vi "Cluster Terminal Get Elements Info.vi"(7 "skip first typedef?":bool, 8 "error in (no error)":errorcluster, 10 "ClusterConstant refnum":refnum<vi>, 11 "Terminal in":refnum<vi>) -> (0 "error out":errorcluster, 1 "is typedef?":bool, 2 "Cluster elements datatypes":string[](array[string]), 3 "Cluster elements names":string[](array[string]), 4 "typedef name":string)   [LabVIEW 2014]
doc: "Return info about cluster elements, as input use Terminal or ClusterConstant (use just one of them)\nIf wired Cluster Constant refnum returns names and datatypes of elements inside cluster. If elemnet has no label, it's returned default name \"item0\" or \"item1\" or ... \"itemN\" which will be also used in generated code.\nIf wired Terminal then is used to get names and datatypes of cluster, it will programmaticaly creates cluster constant on diagram, inspects its elements, removes it and return elements info."
uses:
  TranscriptorBasicObject.lvclass
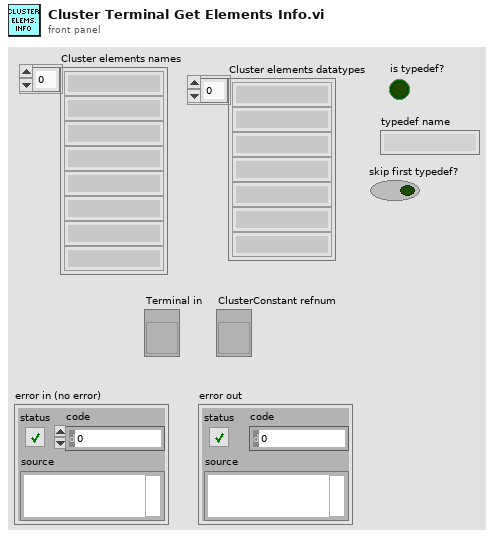
[diagram p1: front panel]
types:
  T1 = enum32{"not a typedef", "typedef", "strict typedef", "class private data"}[]
  T2 = enum32{"not a typedef", "typedef", "strict typedef", "class private data"}
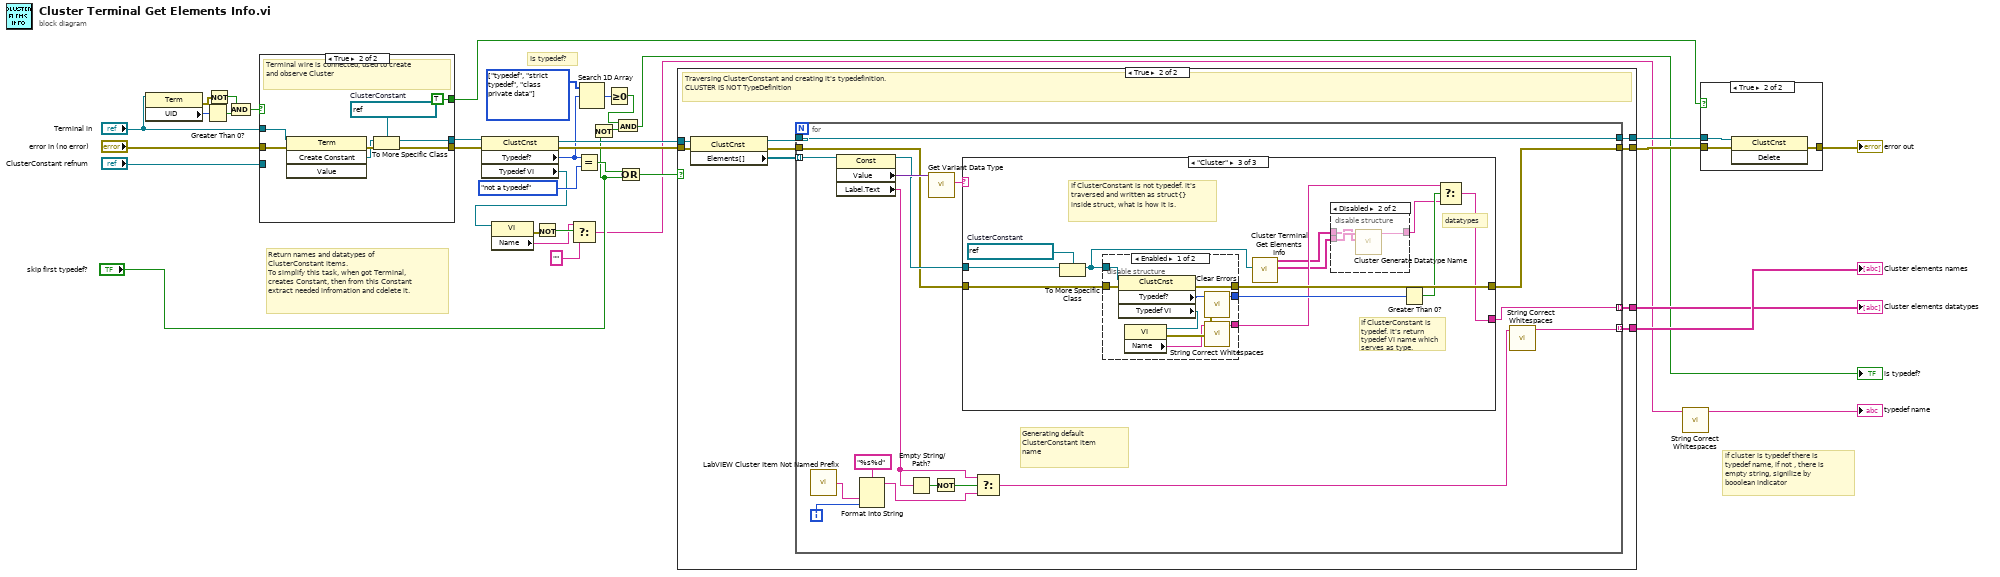
[diagram p0: block diagram]
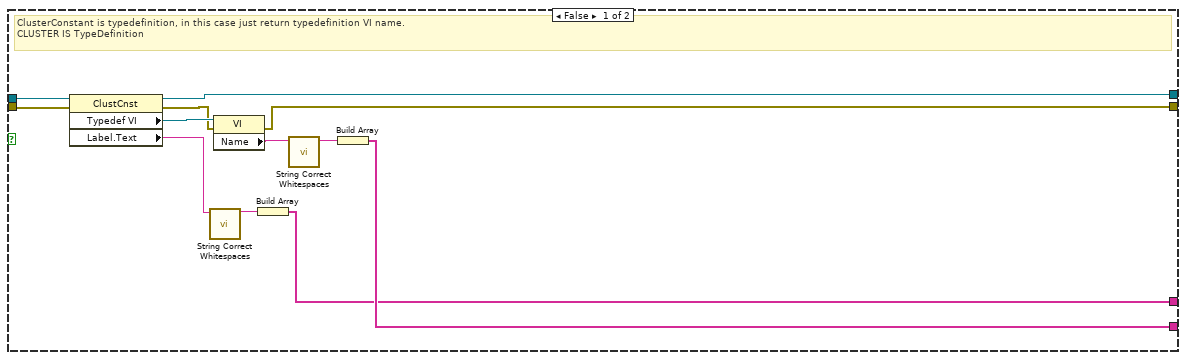
[diagram p2: hidden frame]
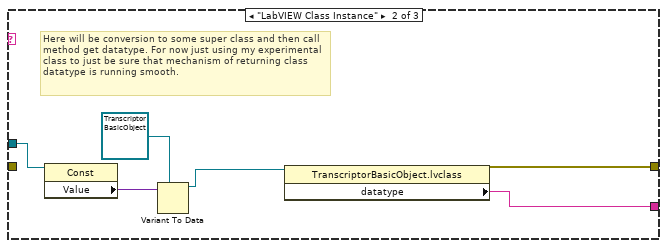
[diagram p4: hidden frame]
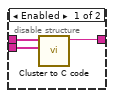
[diagram p5: hidden frame]
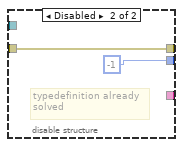
[diagram p6: hidden frame]
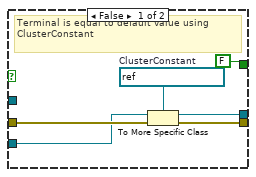
[diagram p8: hidden frame]
diagram:
  w16 = T1 [enum."typedef", enum."strict typedef", enum."class private data"] items=["not a typedef", "typedef", "strict typedef", "class private data"]
  # "if cluster is typedef there is typedef name, if not , there is empty string, signilize by booolean indicator"
  # "Is typedef?"
  # "Return names and datatypes of ClusterConstant items.\nTo simplify this task, when got Terminal, creates Constant, then from this Constant extract needed infromation and cdelete it."
  n1 = property class="Term"(reference="Terminal in") -> (error out=w20:errorcluster, "UID"=w22:i32)  [unwired: 1 in, 1 out]
  n2 = Greater Than 0?(x=w22) -> (x > 0?=w21:bool)
  n3 = Not(x=w20) -> (.not. x?=w19:bool)
  n4 = And(x=w19, y=w21) -> (x .and. y?=w18:bool)
  n5 = case shown="True" w18 {
    tunnel: [w39 w49] -> w28
    tunnel: "error in (no error)" -> [w38 w47]
    tunnel: [w40 w45] -> w29
    tunnel: "Terminal in" -> [_ w43]
    tunnel: [FALSE TRUE] -> w25
    tunnel: "ClusterConstant refnum" -> [w36 _]
    frame False {
      w41 = refnum<vi> refnum  # ClusterConstant
      # "Terminal is equal to default value using ClusterConstant"
      n6 = To More Specific Class(target class=w41, reference=w36, error in=w38) -> (specific class reference=w40:refnum<vi>, error out=w39:errorcluster)
    }
    frame True {
      w44 = refnum<vi> refnum  # ClusterConstant
      # "Terminal wire is connected, used to create and observe Cluster"
      n7 = invoke on="Invoke Node" class="Term" method="Create Constant"(reference=w43, error in=w47) -> (error out=w48:errorcluster, "Create Constant"=w46:refnum<vi>)  [unwired: 2 in, 2 out]
      n8 = To More Specific Class(target class=w44, reference=w46, error in=w48) -> (specific class reference=w45:refnum<vi>, error out=w49:errorcluster)
    }
  }
  n9 = property on="Property Node" class="ClustCnst"(reference=w29, error in=w28) -> (reference out=w27:refnum<vi>, error out=w26:errorcluster, "Typedef?"=w15:T2, "Typedef VI"=w7:refnum<vi>)
  n10 = property on="Property Node" class="VI"(reference=w7) -> (error out=w6:errorcluster, "Name"=w4:string)  [unwired: 1 in, 1 out]
  n11 = Not(x=w6) -> (.not. x?=w5:bool)
  n12 = Select(t=w4, s=w5, f="") -> (s? t:f=w2:string)
  n13 = Equal?(x=w15, y=T2."not a typedef" ("Is Typedef?")) -> (x = y?=w13:bool)
  n14 = Search 1D Array(1D array=w16, element=w15) -> (index of element=w14:i32)  [unwired: 1 in]
  n15 = Not(x="skip first typedef?") -> (.not. x?=w8:bool)
  n16 = Greater Or Equal To 0?(x=w14) -> (x >= 0?=w11:bool)
  n17 = And(x=w11, y=w8) -> (x .and. y?=→"is typedef?":bool)
  n18 = Or(x=w13, y="skip first typedef?") -> (x .or. y?=w12:bool)
  n19 = case shown="True" w12 {
    tunnel: [w55 w70] -> w34
    tunnel: w26 -> [w60 w68]
    tunnel: w27 -> [w61 w66]
    tunnel: [w57 w64] -> w32
    tunnel: [w53 w63] -> w31
    tunnel: [w52 w62] -> w30
    frame False {
      # "ClusterConstant is typedefinition, in this case just return typedefinition VI name.\nCLUSTER IS TypeDefinition"
      n20 = property on="Property Node" class="ClustCnst"(reference=w61, error in=w60) -> (reference out=w57:refnum<vi>, error out=w56:errorcluster, "Typedef VI"=w59:refnum<vi>, "Label.Text"=w51:string)
      n21 = call "String Correct Whitespaces.vi"("String in"=w51) -> ("String out"=w50:string)  [unwired: 10 in]
      n22 = property on="Property Node" class="VI"(reference=w59, error in=w56) -> (error out=w55:errorcluster, "Name"=w58:string)  [unwired: 1 out]
      n23 = Build Array(w50) -> (w52:string[])
      n24 = call "String Correct Whitespaces.vi"("String in"=w58) -> ("String out"=w54:string)  [unwired: 10 in]
      n25 = Build Array(w54) -> (w53:string[])
    }
    frame True {
      # "Traversing ClusterConstant and creating it's typedefinition.\nCLUSTER IS NOT TypeDefinition"
      n26 = property on="Property Node" class="ClustCnst"(reference=w66, error in=w68) -> (reference out=w65:refnum<vi>, error out=w69:errorcluster, "Elements[]"=w67:refnum<vi>[])
      n27 = for {
        tunnel: w67 -> [w87] mode=indexing
        tunnel: w69 -> [w71]
        tunnel: [w73] -> w70
        tunnel: w65 -> [w79]
        tunnel: [w79] -> w64
        tunnel: [w72] -> w62 mode=indexing
        tunnel: [w78] -> w63 mode=indexing
        i -> [w82]
        # "Generating default ClusterConstant item name"
        n28 = call "LabVIEW Cluster Item Not Named Prefix.vi"() -> ("not named cluster item prefix"=w81:string)
        n29 = property class="Const"(reference=w87) -> (reference out=w74:refnum<vi>, "Value"=w75:variant, "Label.Text"=w80:string)  [unwired: 1 in, 1 out]
        n30 = Format Into String(format string="%s%d", w81, w82) -> (resulting string=w83:string)  [unwired: 2 in, 1 out]
        n31 = Empty String/Path?(string/path=w80) -> (empty?=w86:bool)
        n32 = call "Get Variant Data Type.vi"("Variant in"=w75) -> ("first data type"=w76:string)  [unwired: 9 in, 1 out]
        n33 = Not(x=w86) -> (.not. x?=w85:bool)
        n34 = case shown="\"Cluster\"" w76 {
          selector: w76 -> [w88 _ _]
          tunnel: w74 -> [_ w93 w96]
          tunnel: w71 -> [w89 _ w106]
          tunnel: [w89 w94 w104] -> w73
          tunnel: [w88 w95 w103] -> w72
          frame Default {
          }
          frame "LabVIEW Class Instance" {
            # "Here will be conversion to some super class and then call method get datatype. For now just using my experimental class to just be sure that mechanism of returning class datatype is running smooth."
            n35 = property class="Const"(reference=w93) -> ("Value"=w92:variant)  [unwired: 1 in, 2 out]
            n36 = Variant To Data(type=refnum<class "TranscriptorBasicObject.lvclass"> refnum ("TranscriptorBasicObject.lvclass"), Variant=w92) -> (data=w91:refnum<class "TranscriptorBasicObject.lvclass">)  [unwired: 1 in, 1 out]
            n37 = property class="TranscriptorBasicObject.lvclass"(reference=w91) -> (error out=w94:errorcluster, "datatype"=w95:string)  [unwired: 1 in, 1 out]
          }
          frame "Cluster" {
            w107 = refnum<vi> refnum  # ClusterConstant
            # "If ClusterConstant is typedef. it's return typedef VI name which serves as type."
            # "If ClusterConstant is not typedef. it's traversed and written as struct{} inside struct, what is how it is."
            # "datatypes"
            n38 = To More Specific Class(target class=w107, reference=w96) -> (specific class reference=w97:refnum<vi>)  [unwired: 1 in, 1 out]
            n39 = disable-structure shown="Enabled" {
              disable-tunnel: w106 -> [w121 w123]
              disable-tunnel: [w120 -1] -> w105
              disable-tunnel: [w116 w123] -> w104
              disable-tunnel: [w115 _] -> w101
              disable-tunnel: w97 -> [w114 _]
              frame Enabled {
                n40 = property class="ClustCnst"(reference=w114, error in=w121) -> (error out=w116:errorcluster, "Typedef?"=w120:T2, "Typedef VI"=w117:refnum<vi>)  [unwired: 1 out]
                n41 = property class="VI"(reference=w117) -> (error out=w119:errorcluster, "Name"=w118:string)  [unwired: 1 in, 1 out]
                n42 = call <vilib>:"Clear Errors.vi"("error in (no error)"=w119) -> ()  [unwired: 5 in, 2 out]
                n43 = call "String Correct Whitespaces.vi"("String in"=w118) -> ("String out"=w115:string)  [unwired: 10 in]
              }
              frame Disabled {
                # "typedefinition already\nsolved"
              }
            }
            n44 = call "Cluster Terminal Get Elements Info.vi"("ClusterConstant refnum"=w97) -> ("Cluster elements datatypes"=w99:string[], "Cluster elements names"=w100:string[])  [unwired: 6 in, 3 out]
            n45 = disable-structure shown="Disabled" {
              disable-tunnel: w100 -> [w110 w112]
              disable-tunnel: w99 -> [w109 w113]
              disable-tunnel: [w108 w111] -> w98
              frame Enabled {
                n46 = call "Cluster to C code.vi"("Cluster elements datatypes"=w109, "Cluster elements names"=w110) -> ("C code"=w108:string)  [unwired: 9 in]
              }
              frame Disabled {
                n47 = call "Cluster Generate Datatype Name.vi"("Cluster elements names"=w112, "Cluster elements datatypes"=w113) -> ("generated datatype name"=w111:string)  [unwired: 9 in]
              }
            }
            n48 = Greater Than 0?(x=w105) -> (x > 0?=w102:bool)
            n49 = Select(t=w101, s=w102, f=w98) -> (s? t:f=w103:string)
          }
        }
        n50 = Select(t=w80, s=w85, f=w83) -> (s? t:f=w77:string)
        n51 = call "String Correct Whitespaces.vi"("String in"=w77) -> ("String out"=w78:string)  [unwired: 10 in]
      }
    }
  }
  "Cluster elements datatypes" <- w30
  "Cluster elements names" <- w31
  n52 = call "String Correct Whitespaces.vi"("String in"=w2) -> ("String out"=→"typedef name":string)  [unwired: 10 in]
  n53 = case shown="True" w25 {
    tunnel: [w124 w127] -> w35
    tunnel: w34 -> [w124 w126]
    tunnel: w32 -> [_ w125]
    frame False {
    }
    frame True {
      n54 = invoke on="Invoke Node" class="ClustCnst" method="Delete"(reference=w125, error in=w126) -> (error out=w127:errorcluster)  [unwired: 1 in, 2 out]
    }
  }
  "error out" <- w35
